vi "April Tag Image AE 3.vi"(10 "Camera Name":string, 11 "Apriltag Image in":T1(plugin-control)) -> (3 "Apriltag Image out":T1(plugin-control))   [LabVIEW 2025]
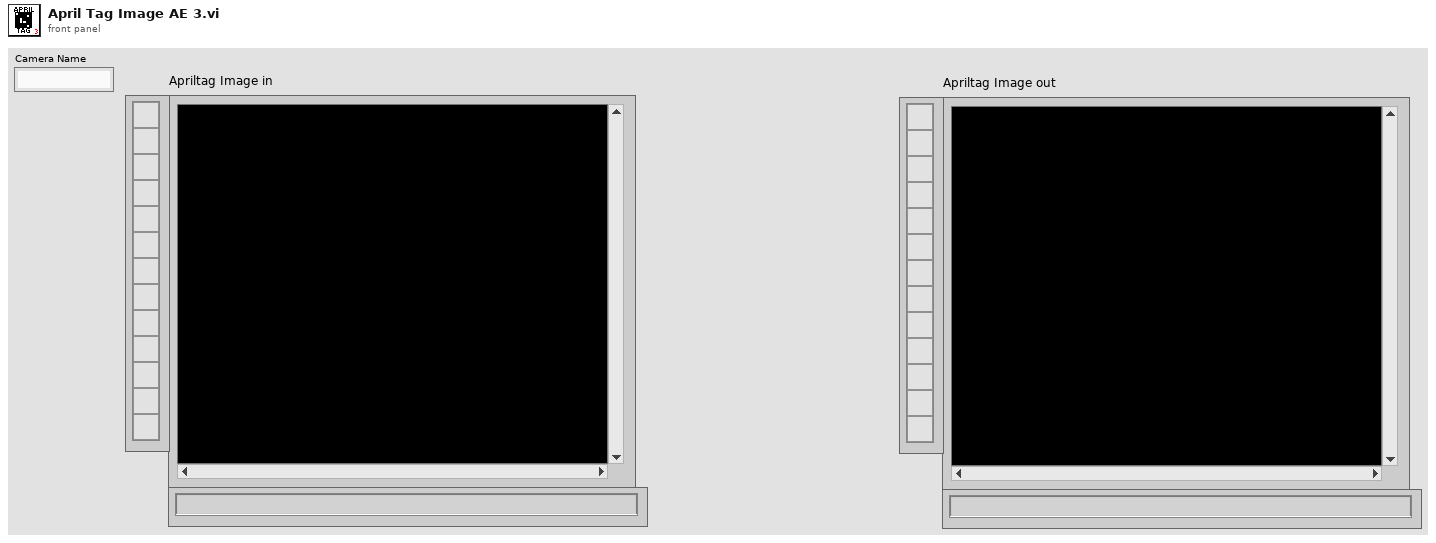
[diagram p1: front panel]
types:
  T1 = typedef "IMAQ Image.ctl" = refnum<image>
  T2 = typedef "Image Type" = u32
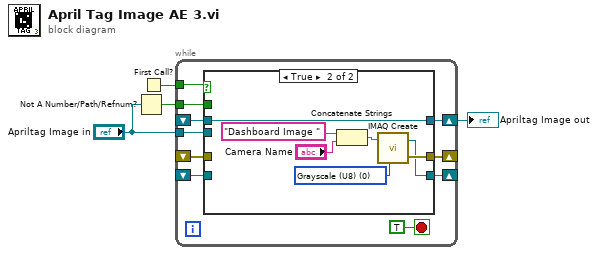
[diagram p0: block diagram]
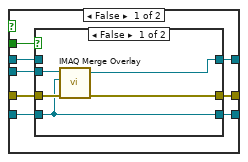
[diagram p2: hidden frame]
diagram:
  n1 = Not A Number/Path/Refnum?(number/path/refnum="Apriltag Image in") -> (NaN/Path/Refnum?=w3:bool)
  n2 = First Call?() -> (First Call?: T/F=w4:bool)
  n3 = while {
    tunnel: w3 -> [w14]
    tunnel: "Apriltag Image in" -> [w13]
    shift-right: [w12] -> w1
    shift-left: _ -> [w11]
    shift-right: [w7] -> _
    shift-left: _ -> [w9]
    tunnel: w4 -> [w6]
    shift-right: [w5] -> _
    shift-left: _ -> [w8]
    stop <- TRUE stop-if-true
    n4 = case shown="True" w6 {
      tunnel: w14 -> [w22 _]
      tunnel: w13 -> [w21 _]
      tunnel: [w20 w32] -> w12
      tunnel: w11 -> [w19 w32]
      tunnel: w9 -> [w18 _]
      tunnel: w8 -> [w17 _]
      tunnel: [w16 w34] -> w7
      tunnel: [w15 w33] -> w5
      frame False {
        n5 = case shown="False" w22 {
          tunnel: w21 -> [w27 _]
          tunnel: [w25 w30] -> w20
          tunnel: w19 -> [_ w30]
          tunnel: w18 -> [w26 w29]
          tunnel: w17 -> [w23 w28]
          tunnel: [w24 w29] -> w16
          tunnel: [w23 w28] -> w15
          frame False {
            n6 = call "IMAQ Merge Overlay"("error in (no error)"=w26, "Image Dst"=w23, "Image Src"=w27) -> ("error out"=w24:errorcluster, "Image Dst Out"=w25:T1)  [unwired: 7 in]
          }
          frame True {
          }
        }
      }
      frame True {
        w36 = T2 0 items=["Grayscale (U8)", "Grayscale (I16)", "Grayscale (SGL)", "Complex (CSG)", "RGB (U32)", "HSL (U32)", "RGB (U64)", "Grayscale (U16)"] ("Image Type")
        n7 = Concatenate Strings("Dashboard Image " ("string"), "Camera Name") -> (w35:string)
        n8 = call "IMAQ Create"("Image Name"=w35, "Image Type"=w36) -> ("New Image"=w33:T1, "error out"=w34:errorcluster)  [unwired: 2 in, 1 out]
      }
    }
  }
  "Apriltag Image out" <- w1
